vi "initialize.vi"   [LabVIEW 2015, in "lv-graph-global.lvlib"]
doc: "This polymorphic VI provides access to two initialize methods, once that provides data (and infers the configuration from it) and the other that provides the configuration directly."
uses:
  lv-graph-global.lvlib
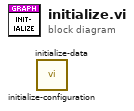
[diagram p0: block diagram]
diagram:
  n1 = call "initialize-configuration.vi"() -> ()  [unwired: 10 in, 2 out]
  n2 = call "initialize-data.vi"() -> ()  [unwired: 10 in, 2 out]
